vi "Listen.vi"(8 "error in (no error)":errorcluster, 11 "Debug Message Receiver in":refnum<class "Debug Message Receiver.lvclass">) -> (0 "error out":errorcluster, 3 "Debug Message Receiver out":refnum<class "Debug Message Receiver.lvclass">)   [LabVIEW 2020, in "Debug Message Receiver.lvclass"]
uses:
  Debug Message Receiver.lvclass
  C:/Users/anton/Documents/GitHub/triarc-debugger/source/Process/Debug Process.lvclass
  Process/Debug Process.lvclass/Debug Process.ctl
  Process/Public/Lifecycle/Get Lifecycle State.vi
  <vilib>/Utility/error.llb/Clear Errors.vi
  <vilib>/Utility/error.llb/Error Cluster From Error Code.vi
  Process/Debug Process.lvclass
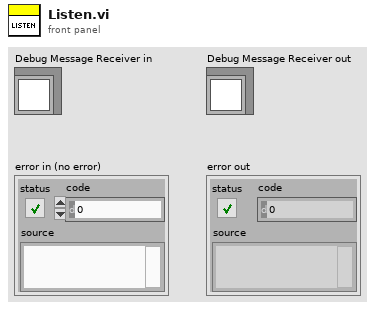
[diagram p1: front panel]
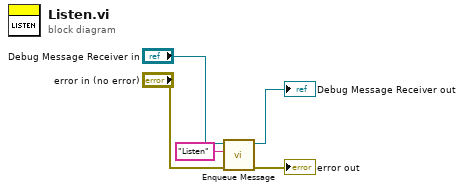
[diagram p0: block diagram]
diagram:
  n1 = call "Enqueue Message.vi"("error in (no error)"="error in (no error)", "Message"="Listen", "Process In"="Debug Message Receiver in") -> ("error out"=→"error out":errorcluster, "Process Out"=→"Debug Message Receiver out":refnum<class "Debug Message Receiver.lvclass">)  [unwired: 7 in]
